vi "phase_three.vi"   [LabVIEW 2015]
uses:
  <vilib>/NXT/Block Support/NXT_OutputPort.ctl
  all_done?.vi
  <vilib>/NXT/Dual Mode Library/Sound/PlayC.vi
  <vilib>/NXT/Dual Mode Library/Waits/Wait_Num.vi
  <vilib>/NXT/NXTIO Xnodes/NXTIONodeSubVIs/NXTMotorRunDistance.vi
  <vilib>/NXT/NXTIO Xnodes/AddressXNode/NXTIOAddress.xnode
  <vilib>/NXT/NXTIO Xnodes/NXTIOXNode/NXTIO.xnode
  <vilib>/NXT/Subs/LVHSConnector.ctl
  <vilib>/NXT/LegoClasses/BrickReference/BrickReference.lvclass
types:
  T1 = typedef "LVHSConnector.ctl" = refnum<class "BrickReference.lvclass">
  T2 = typedef "NXT_OutputPort.ctl" = u8
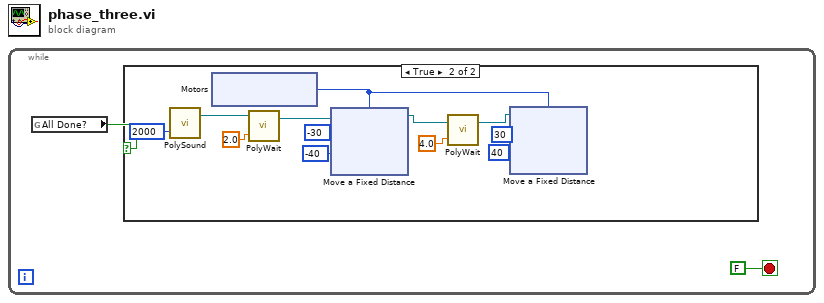
[diagram p0: block diagram]
diagram:
  n1 = while {
    stop <- FALSE stop-if-true
    n2 = global read "all_done?.vi" "All Done?"() -> (w1:bool)
    n3 = case shown="True" w1 {
      frame False {
      }
      frame True {
        n4 = call-poly <vilib>:"PolySound.vi"("Duration (500 ms)"=u16 2000) -> ("NXT/EV3"=w14:T1)  [unwired: 3 in]
        n5 = xnode "Motors"() -> ("Motor"=w3:T2)
        n6 = call-poly <vilib>:"PolyWait.vi"("Time (1 sec)"=sgl 2.0, "NXT/EV3"=w14) -> ("NXT/EV3"=w12:T1)  [unwired: 2 in]
        n7 = xnode "Move a Fixed Distance"("Speed 1"=i8 -40, "Distance 1"=-30, "Motors"=w3, "NXT/EV3"=w12) -> ("NXT/EV3"=w7:T1)
        n8 = call-poly <vilib>:"PolyWait.vi"("Time (1 sec)"=sgl 4.0, "NXT/EV3"=w7) -> ("NXT/EV3"=w8:T1)  [unwired: 2 in]
        n9 = xnode "Move a Fixed Distance"("Speed 1"=i8 40, "Distance 1"=30, "Motors"=w3, "NXT/EV3"=w8) -> ()  [unwired: 1 out]
      }
    }
  }
